vi "Begin.vi"(8 "error in":errorcluster) -> (0 "error out":errorcluster)   [LabVIEW 2019]
doc: "Called before other user functions, this VI is expected to open initial I/O refnums, load in file data, and do all program initialization. Notice that the <B>error out</B> terminal is simply used for data flow. Wiring it to other structures or subVIs ensures that this VI runs first."
uses:
  <vilib>/Rock Robotics/WPI/DriverStation/WPI_DriverStationRobotMode2.ctl
  <vilib>/Rock Robotics/WPI/Joystick/WPI_JoystickDeviceEnum.ctl
  <vilib>/Rock Robotics/SystemInterfaces/DIO/FPGA_DIOPWMChannel.ctl
  <vilib>/Rock Robotics/SystemInterfaces/i2clib/i2c_bus.ctl
  <vilib>/Rock Robotics/WPI/SafetyOutput/WPI_SafetyOutputConfigMenu.ctl
  <vilib>/Rock Robotics/SystemInterfaces/AI/FPGA_AIGyroChannel.ctl
  <vilib>/Rock Robotics/SystemInterfaces/DIO/FPGA_DIOChannel.ctl
  Robot Global Data.vi
  <vilib>/Rock Robotics/Network Tables/NT Write String Array.vi
  <vilib>/Rock Robotics/WPI/MotorControl/WPI_MotorControlOpen VictorSP.vi
  <vilib>/Rock Robotics/WPI/RobotDrive/WPI_RobotDriveOpen2MotorWithVictorSP.vi
  <vilib>/Rock Robotics/WPI/Gyro/WPI_GyroAnalogOpen.vi
  <vilib>/Rock Robotics/WPI/MotorControl/WPI_MotorControlOpen SPARK.vi
  <vilib>/Rock Robotics/WPI/Switch/WPI_SwitchOpenLimit.vi
  <vilib>/Rock Robotics/WPI/RobotDrive/WPI_RobotDriveOpen2MotorWithSPARK.vi
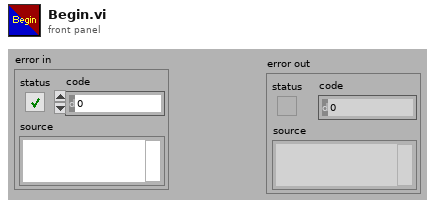
[diagram p1: front panel]
types:
  T1 = typedef "FPGA_DIOPWMChannel.ctl" = enum8{"PWM 0", "PWM 1", "PWM 2", "PWM 3", "PWM 4", "PWM 5", "PWM 6", "PWM 7", "PWM 8", "PWM 9", "PWM MXP 0", "PWM MXP 1", "PWM MXP 2", "PWM MXP 3", "PWM MXP 4", "PWM MXP 5", "PWM MXP 6", "PWM MXP 7", "PWM MXP 8", "PWM MXP 9", "Invalid"}
  T2 = typedef "FPGA_DIOChannel.ctl" = enum8{"DIO 0", "DIO 1", "DIO 2", "DIO 3", "DIO 4", "DIO 5", "DIO 6", "DIO 7", "DIO 8", "DIO 9", "DIO MXP 0", "DIO MXP 1", "DIO MXP 2", "DIO MXP 3", "DIO MXP 4", "DIO MXP 5", "DIO MXP 6", "DIO MXP 7", "DIO MXP 8", "DIO MXP 9", "DIO MXP 10", "DIO MXP 11", "DIO MXP 12", "DIO MXP 13", "DIO MXP 14", "DIO MXP 15", "SPI Port CS1", "SPI Port CS2", "SPI Port CS3", "SPI Port MISO", "SPI Port MOSI", "Invalid"}
  T3 = typedef "FPGA_AIGyroChannel.ctl" = enum8{"AI 0", "AI 1", "Invalid"}
  T4 = typedef "WPI_SafetyOutputConfigMenu.ctl" = enum16{"Enable", "Disable"}
  T5 = typedef "i2c_bus.ctl" = enum16{"I2C On-Board", "I2C MXP", "Invalid"}
  T6 = typedef "WPI_JoystickDeviceEnum.ctl" = enum16{"USB 0", "USB 1", "USB 2", "USB 3", "USB 4", "USB 5"}
  T7 = typedef "WPI_DriverStationRobotMode2.ctl" = enum16{"Autonomous Disabled", "Autonomous Enabled", "Teleop Disabled", "Teleop Enabled", "Disconnected", "Finish", "Test Disabled", "Test Enabled", "Emergency Stopped"}
  T8 = typedef "WPI_GyroDevRef.ctl" = cluster{"DevStatus":errorcluster, "Analog Channel":T9, "Gain (VoltsPerDegree/Second)":dbl, "Gyro Type":enum16{"Analog", "XRS450"}, "Handle":i32, "SPI Bus":T10, "Device Found":bool, "Sample Rate":dbl, "Calibrate On Open":bool, "Offset":dbl}
  T9 = typedef "FPGA_AIChannel.ctl" = enum8{"AI 0", "AI 1", "AI 2", "AI 3", "AI MXP 0", "AI MXP 1", "AI MXP 2", "AI MXP 3", "Invalid"}
  T10 = typedef "spi_bus.ctl" = enum16{"SPI On-Board, CS0", "SPI On-Board, CS1", "SPI On-Board, CS2", "SPI On-Board, CS3", "SPI MXP", "Invalid"}
  T11 = typedef "WPI_MotorControlDeviceRef.ctl" = cluster{"DeviceStatus":errorcluster, "Type":T12, "PWM":cluster{"PWM Channel":T1, "DeadBand":T13}, "CAN":cluster{"Device Number":u8, "SetOutput VI Ref":variant, "GetOutput VI Ref":variant, "Enable VI Ref":variant, "Disable VI Ref":variant, "Data":variant}, "Invert":bool, "DIO PWM":cluster{"PWM \"Enable\" Channel":T1, "DIOChannel":T2, "PWM Rate":dbl}}
  T12 = typedef "WPI_MotorControlType.ctl" = enum16{"PWM", "CAN", "DIO PWM"}
  T13 = typedef "WPI_PWMDeadband.ctl" = cluster{"Name":string, "maxPositivePwm":i32, "minPositivePwm":i32, "centerPwm":i32, "maxNegativePwm":i32, "minNegativePwm":i32, "angularRange":u16}
  T14 = typedef "WPI_JoystickDevRef.ctl" = cluster{"Device":T6}
  T15 = typedef "Color Sensor V3 DevRef.ctl" = cluster{"I2CDevRef":T16}
  T16 = typedef "WPI_I2CDevRef.ctl" = cluster{"DevStatus":errorcluster, "Device Address":u8, "Handle":i32, "I2C Bus":T5}
  T17 = typedef "WPI_RobotDriveDevRef.ctl" = cluster{"DevStatus":errorcluster, "Motors[]":T11[], "Square Inputs":bool, "Max Output":dbl}
  T18 = typedef "WPI_SwitchDevRef.ctl" = cluster{"DevStatus":errorcluster, "DIO Channel":T2, "CntIndex":T19, "Normally Closed":bool}
  T19 = typedef "FPGA_CounterCtrSystemIndex.ctl" = enum8{"Ctr 0", "Ctr 1", "Ctr 2", "Ctr 3", "Ctr 4", "Ctr 5", "Ctr 6", "Ctr 7", "Invalid"}
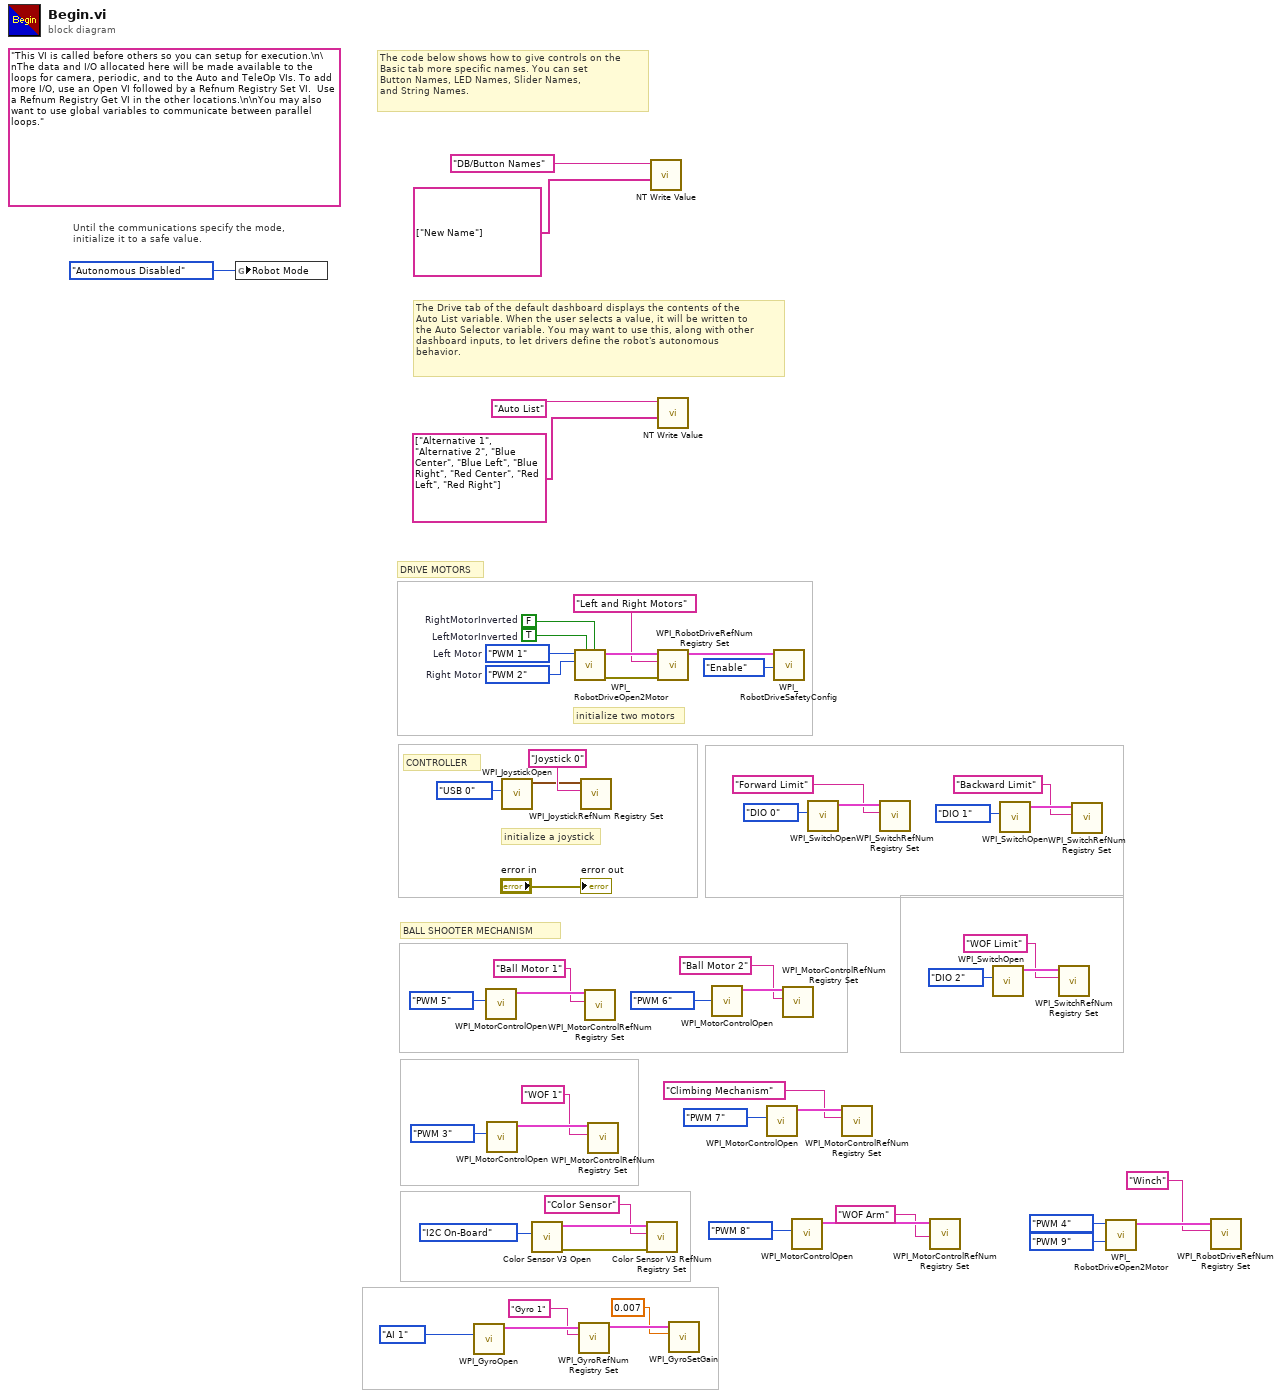
[diagram p0: block diagram]
diagram:
  w31 = FPGA_DIOPWMChannel."PWM 2"  # Right Motor
  w32 = FPGA_DIOPWMChannel."PWM 1"  # Left Motor
  w36 = TRUE  # LeftMotorInverted
  w37 = FALSE  # RightMotorInverted
  (unwired) "This VI is called before others so you can setup for execution.\n\nThe data and I/O allocated here will be made available to the loops for camera, periodic, and to the Auto and TeleOp VIs. To add more I/O, use an Open VI followed by a Refnum Registry Set VI.  Use a Refnum Registry Get VI in the other locations.\n\nYou may also want to use global variables to communicate between parallel loops."
  # "DRIVE MOTORS"
  # "initialize two motors"
  # "CONTROLLER"
  # "BALL SHOOTER MECHANISM"
  # "The Drive tab of the default dashboard displays the contents of the\nAuto List variable. When the user selects a value, it will be written to\nthe Auto Selector variable. You may want to use this, along with other\ndashboard inputs, to let drivers define the robot's autonomous\nbehavior."
  # "The code below shows how to give controls on the\nBasic tab more specific names. You can set\nButton Names, LED Names, Slider Names,\nand String Names."
  # "initialize a joystick"
  # "Until the communications specify the mode,\ninitialize it to a safe value."
  n1 = global write "Robot Global Data.vi" "Robot Mode"(WPI_DriverStationRobotMode2."Autonomous Disabled" ("Robot Mode")) -> ()
  n2 = call-poly <vilib>:"WPI_GyroOpen.vi"("Analog Channel"=FPGA_AIGyroChannel."AI 1") -> ("GyroDevRef"=w27:T8)  [unwired: 8 in, 2 out]
  n3 = call-poly <vilib>:"WPI_MotorControlOpen.vi"("PWM Channel"=FPGA_DIOPWMChannel."PWM 5") -> ("MotorControlDeviceRef"=w47:T11)  [unwired: 9 in, 1 out]
  n4 = call-poly <vilib>:"WPI_MotorControlOpen.vi"("PWM Channel"=FPGA_DIOPWMChannel."PWM 3") -> ("MotorControlDeviceRef"=w44:T11)  [unwired: 9 in, 1 out]
  n5 = call <vilib>:"WPI_JoystickOpen.vi"("JoystickDevice"=WPI_JoystickDeviceEnum."USB 0") -> ("JoystickDevRef"=w53:T14)  [unwired: 10 in]
  n6 = call <vilib>:"Color Sensor V3 Open.vi"("I2C Bus"=i2c_bus."I2C On-Board") -> ("error out"=w39:errorcluster, "ColorSensorDevRef"=w41:T15)  [unwired: 9 in]
  n7 = call-poly <vilib>:"WPI_RobotDriveOpen2Motor.vi"("Right Motor Inverted"=w37, "Left Motor Inverted"=w36, "Right Motor"=w31, "Left Motor"=w32) -> ("error out"=w33:errorcluster, "RobotDriveDevRef"=w35:T17)  [unwired: 1 in, 5 out]
  n8 = call <vilib>:"WPI_GyroRefNum Registry Set.vi"("refnum name"="Gyro 1", "GyroDevRef"=w27) -> ("GyroDevRef"=w24:T8)  [unwired: 8 in, 1 out]
  n9 = call <vilib>:"WPI_JoystickRefNum Registry Set.vi"("refnum name"="Joystick 0", "JoystickDevRef"=w53) -> ()  [unwired: 8 in, 2 out]
  n10 = call <vilib>:"WPI_MotorControlRefNum Registry Set.vi"("refnum name"="Ball Motor 1", "MotorControlDevRef"=w47) -> ()  [unwired: 8 in, 2 out]
  n11 = call <vilib>:"WPI_MotorControlRefNum Registry Set.vi"("refnum name"="WOF 1", "MotorControlDevRef"=w44) -> ()  [unwired: 8 in, 2 out]
  n12 = call <vilib>:"Color Sensor V3 RefNum Registry Set.vi"("error in (no error)"=w39, "refnum name"="Color Sensor", "ColorSensorDevRef"=w41) -> ()  [unwired: 7 in, 2 out]
  n13 = call-poly <vilib>:"NT Write Value.vi"("String Array"=string[] ["New Name"], "Name"="DB/Button Names") -> ()  [unwired: 9 in, 1 out]
  n14 = call-poly <vilib>:"NT Write Value.vi"("String Array"=string[] ["Alternative 1", "Alternative 2", "Blue Center", "Blue Left", "Blue Right", "Red Center", "Red Left", "Red Right"], "Name"="Auto List") -> ()  [unwired: 9 in, 1 out]
  n15 = call <vilib>:"WPI_RobotDriveRefNum Registry Set.vi"("error in (no error)"=w33, "refnum name"="Left and Right Motors", "RobotDriveDevRef"=w35) -> ("RobotDriveDevRef"=w30:T17)  [unwired: 1 in, 7 out]
  n16 = call <vilib>:"WPI_GyroSetGain.vi"("Gain (VoltsPerDegree/Second)"=0.007, "GyroDevRef"=w24) -> ()  [unwired: 8 in, 2 out]
  n17 = call-poly <vilib>:"WPI_MotorControlOpen.vi"("PWM Channel"=FPGA_DIOPWMChannel."PWM 6") -> ("MotorControlDeviceRef"=w22:T11)  [unwired: 9 in, 1 out]
  n18 = call-poly <vilib>:"WPI_MotorControlOpen.vi"("PWM Channel"=FPGA_DIOPWMChannel."PWM 7") -> ("MotorControlDeviceRef"=w9:T11)  [unwired: 9 in, 1 out]
  n19 = call <vilib>:"WPI_RobotDriveSafetyConfig.vi"("mode"=WPI_SafetyOutputConfigMenu."Enable", "RobotDriveDevRef"=w30) -> ()  [unwired: 8 in, 2 out]
  n20 = call <vilib>:"WPI_MotorControlRefNum Registry Set.vi"("refnum name"="Ball Motor 2", "MotorControlDevRef"=w22) -> ()  [unwired: 8 in, 2 out]
  n21 = call-poly <vilib>:"WPI_MotorControlOpen.vi"("PWM Channel"=FPGA_DIOPWMChannel."PWM 8") -> ("MotorControlDeviceRef"=w6:T11)  [unwired: 9 in, 1 out]
  n22 = call-poly <vilib>:"WPI_SwitchOpen.vi"("DIO Channel"=FPGA_DIOChannel."DIO 0") -> ("SwitchDevRef"=w19:T18)  [unwired: 9 in, 1 out]
  n23 = call <vilib>:"WPI_MotorControlRefNum Registry Set.vi"("refnum name"="Climbing Mechanism", "MotorControlDevRef"=w9) -> ()  [unwired: 8 in, 2 out]
  n24 = call <vilib>:"WPI_SwitchRefNum Registry Set.vi"("refnum name"="Forward Limit", "SwitchDevRef"=w19) -> ()  [unwired: 8 in, 2 out]
  n25 = call <vilib>:"WPI_MotorControlRefNum Registry Set.vi"("refnum name"="WOF Arm", "MotorControlDevRef"=w6) -> ()  [unwired: 8 in, 2 out]
  n26 = call-poly <vilib>:"WPI_SwitchOpen.vi"("DIO Channel"=FPGA_DIOChannel."DIO 2") -> ("SwitchDevRef"=w12:T18)  [unwired: 9 in, 1 out]
  n27 = call-poly <vilib>:"WPI_SwitchOpen.vi"("DIO Channel"=FPGA_DIOChannel."DIO 1") -> ("SwitchDevRef"=w16:T18)  [unwired: 9 in, 1 out]
  n28 = call <vilib>:"WPI_SwitchRefNum Registry Set.vi"("refnum name"="WOF Limit", "SwitchDevRef"=w12) -> ()  [unwired: 8 in, 2 out]
  n29 = call <vilib>:"WPI_SwitchRefNum Registry Set.vi"("refnum name"="Backward Limit", "SwitchDevRef"=w16) -> ()  [unwired: 8 in, 2 out]
  n30 = call-poly <vilib>:"WPI_RobotDriveOpen2Motor.vi"("Right Motor"=FPGA_DIOPWMChannel."PWM 9", "Left Motor"=FPGA_DIOPWMChannel."PWM 4") -> ("RobotDriveDevRef"=w2:T17)  [unwired: 8 in, 1 out]
  n31 = call <vilib>:"WPI_RobotDriveRefNum Registry Set.vi"("refnum name"="Winch", "RobotDriveDevRef"=w2) -> ()  [unwired: 8 in, 2 out]
  "error out" <- "error in"
